vi "ExerciceSerrure2.vi"() -> ()   [LabVIEW 2018]
uses:
  Serrure_Var.vi
panel:
  out "?":bool
  in  "?":bool
  out "Tentatives Max":dbl
  out "Tentatives":dbl
  in  "Code 3":i8(knob) min=0 max=9 scale=0.0..9.0
  in  "Code 2":i8(knob) min=0 max=9 scale=0.0..9.0
  in  "Code 1":i8(knob) min=0 max=9 scale=0.0..9.0
  # "/"
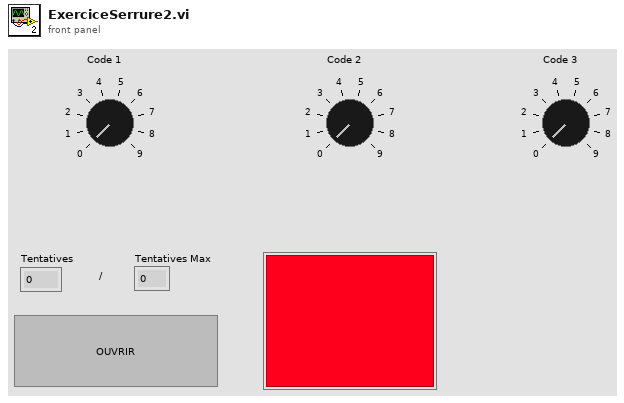
[diagram p1: front panel]
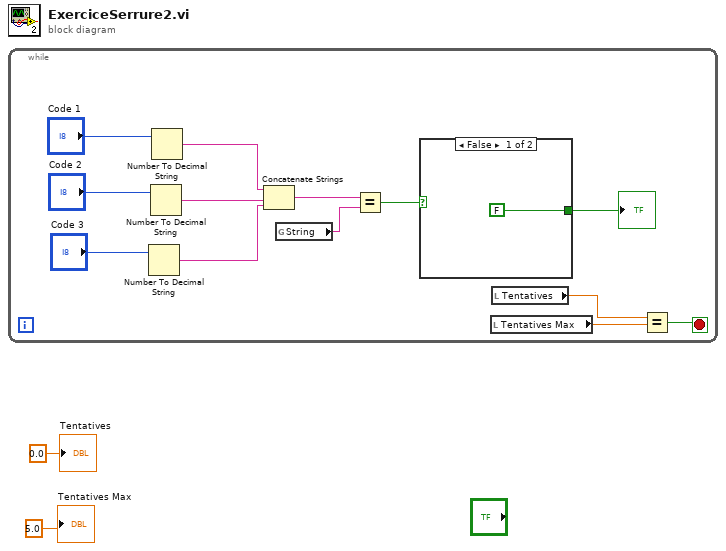
[diagram p0: block diagram]
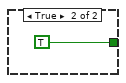
[diagram p2: hidden frame]
diagram:
  n1 = while {
    stop <- w5 stop-if-true
    n2 = Number To Decimal String(number="Code 3") -> (decimal integer string=w10:string)  [unwired: 1 in]
    n3 = Number To Decimal String(number="Code 2") -> (decimal integer string=w11:string)  [unwired: 1 in]
    n4 = Number To Decimal String(number="Code 1") -> (decimal integer string=w12:string)  [unwired: 1 in]
    n5 = Concatenate Strings(w12, w11, w10) -> (w9:string)
    n6 = global read "Serrure_Var.vi" "String"() -> (w8:string)
    n7 = Equal?(x=w9, y=w8) -> (x = y?=w7:bool)
    n8 = case shown="False" w7 {
      tunnel: [FALSE TRUE] -> w6
      frame False {
      }
      frame True {
      }
    }
    "?" <- w6
    n9 = local read "Tentatives Max"() -> (w4:dbl)
    n10 = local read "Tentatives"() -> (w3:dbl)
    n11 = Equal?(x=w3, y=w4) -> (x = y?=w5:bool)
  }
  "Tentatives" <- 0.0 ("Tentatives")
  "Tentatives Max" <- 5.0 ("Tentatives Max")
